vi "single REQ.vi"(8 "error in (no error)":errorcluster, 9 "binary data in":u8[](array[numeric])=[1, 2, 3, 4], 10 "Arguments":T3={"arg1"=1, "arg2"=3.14}, 11 "fun2call":T2) -> (0 "error out":errorcluster, 1 "detailed err description or other information":string, 2 "parsed response":T1={"bin_lng"=1, "a1"=1, "a2"=3.14}, 4 "roundtrip time":dbl, 5 "short err code":u8)   [LabVIEW 2018, in "LV-Julia_ZMQ-Roundtrip_lib.lvlib"]
uses:
  LV-Julia_ZMQ-Roundtrip_lib.lvlib
  example args cluster.ctl
  Julia functions enum.ctl
  example server response cluster.ctl
  example Fun&args cluster.ctl
  commands LV2Jl.ctl
  Commands v2.ctl
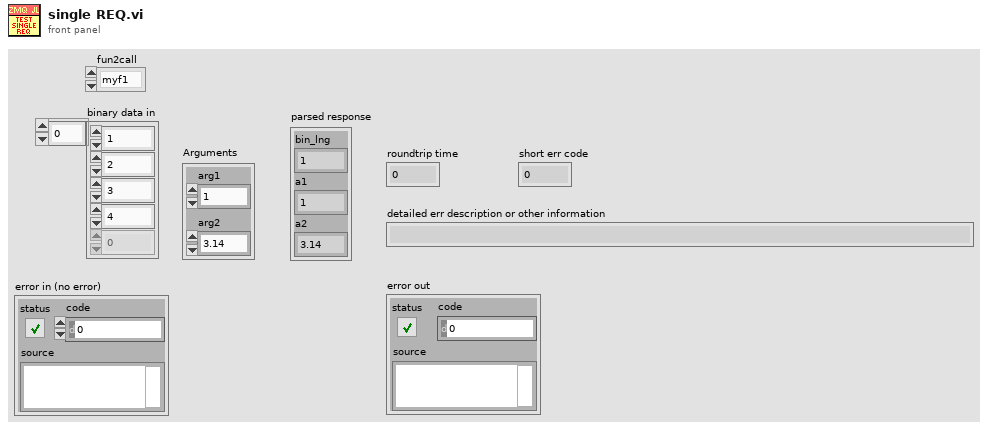
[diagram p1: front panel]
types:
  T1 = typedef "example server response cluster.ctl" = cluster{"bin_lng":i32, "a1":i32, "a2":dbl}
  T2 = typedef "Julia functions enum.ctl" = enum16{"myf1", "myf2", "myf3"}
  T3 = typedef "example args cluster.ctl" = cluster{"arg1":i32, "arg2":dbl}
  T4 = typedef "commands LV2Jl.ctl" = u8
  T5 = typedef "example Fun&args cluster.ctl" = cluster{"fun2call":string, "arg1":i32, "arg2":dbl}
  T6 = typedef "LV-Julia_ZMQ-Roundtrip_lib.lvlib/Commands v2.ctl" = enum16{"Start Jl-server & Init LV-client", "Send request & Get response ", "Stop Jl-server & Cleanup LV-client", "Cleanup LV-client", "Start Jl-server", "Stop Jl-server", "Init LV-Client", "Cleanup LV-Client", "(not allowed)", "Set LV Client state", "Set Jl Server state"}
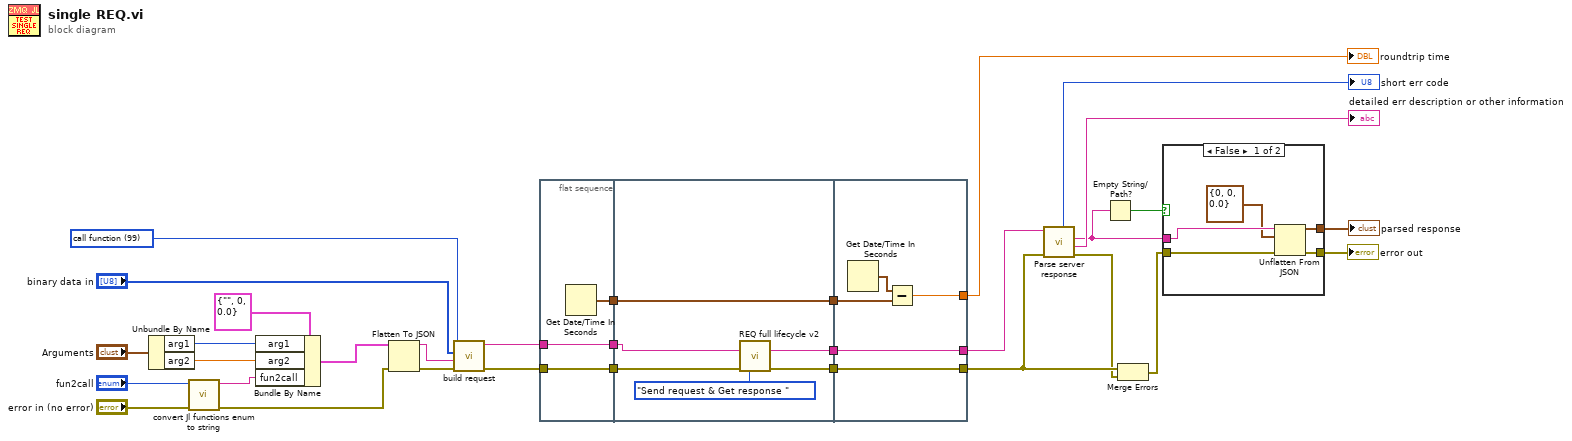
[diagram p0: block diagram]
diagram:
  w18 = T4 99 items=["call function"=99, "ping"=112, "stop"=115] ("Command")
  n1 = Unbundle By Name("Arguments") -> ("arg1"=w13:i32, "arg2"=w14:dbl)
  n2 = call "convert Jl functions enum to string.vi"("error in (no error)"="error in (no error)", "fun2call"="fun2call") -> ("error out"=w10:errorcluster, "String out"=w2:string)  [unwired: 8 in]
  n3 = Bundle By Name(cluster=T5 {"fun2call"="", "arg1"=0, "arg2"=0.0} ("fun and args"), "arg1"=w13, "arg2"=w14, "fun2call"=w2) -> (w12:T5)
  n4 = Flatten To JSON(anything=w12, error in (no error)=w10) -> (JSON string=w11:string, 11:w9:errorcluster)  [unwired: 1 in]
  n5 = call "build request.vi"("error in (no error)"=w9, "JSON data"=w11, "binary data"="binary data in", "Command"=w18) -> ("error out"=w21:errorcluster, "REQ string"=w19:string)  [unwired: 6 in]
  n6 = flat-sequence {
    tunnel: w21 -> [w35]
    tunnel: [w35] -> w26
    tunnel: [w34] -> w25
    tunnel: [w33] -> w20
    tunnel: w19 -> [w33]
    tunnel: [w40] -> w28
    tunnel: [w39] -> w27
    tunnel: w26 -> [w41]
    tunnel: w25 -> [w38]
    tunnel: [w38] -> w24
    tunnel: w20 -> [w37]
    tunnel: [w45] -> w31
    tunnel: [w46] -> w32
    tunnel: w28 -> [w46]
    tunnel: w27 -> [w45]
    tunnel: w24 -> [w43]
    tunnel: [w42] -> w23
    frame #0 {
      n7 = Get Date/Time In Seconds() -> (seconds since 1Jan1904=w34:timestamp)
    }
    frame #1 {
      n8 = call "REQ full lifecycle v2.vi"("data to send"=w37, "error in"=w41, "command"=Commands_v2."Send request & Get response ") -> ("server response"=w40:string, "error out"=w39:errorcluster)  [unwired: 9 in, 2 out]
    }
    frame #2 {
      n9 = Get Date/Time In Seconds() -> (seconds since 1Jan1904=w44:timestamp)
      n10 = Subtract(x=w44, y=w43) -> (x-y=w42:dbl)
    }
  }
  n11 = call "Parse server response.vi"("error in (no error)"=w31, "server response in"=w32) -> ("error out"=w30:errorcluster, "detailed err description"=→"detailed err description or other information":string, "JSON out"=w6:string, "short err code"=→"short err code":u8)  [unwired: 3 in, 3 out]
  n12 = Empty String/Path?(string/path=w6) -> (empty?=w5:bool)
  n13 = Merge Errors(w31, w30) -> (w8:errorcluster)
  n14 = case shown="False" w5 {
    tunnel: w6 -> [w51 _]
    tunnel: w8 -> [w50 w52]
    tunnel: [w49 w52] -> w7
    tunnel: [w48 _] -> w1
    frame False {
      n15 = Unflatten From JSON(JSON string=w51, type and defaults=T1 {"bin_lng"=0, "a1"=0, "a2"=0.0} ("parsed response"), error in (no error)=w50) -> (value=w48:T1, error out=w49:errorcluster)  [unwired: 4 in]
    }
    frame True {
    }
  }
  "error out" <- w7
  "parsed response" <- w1
  "roundtrip time" <- w23
